vi "21.vi"() -> ()   [LabVIEW 2021]
panel:
  out "Numeric":i32
  out "Array":i32[](array[numeric])
  in  "Number":i32
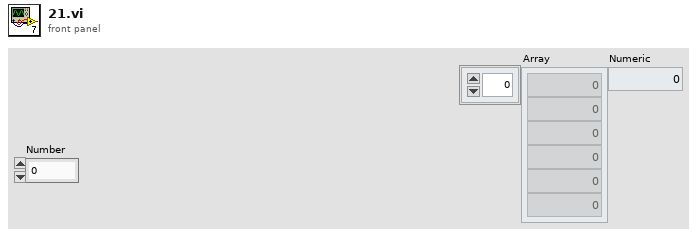
[diagram p1: front panel]
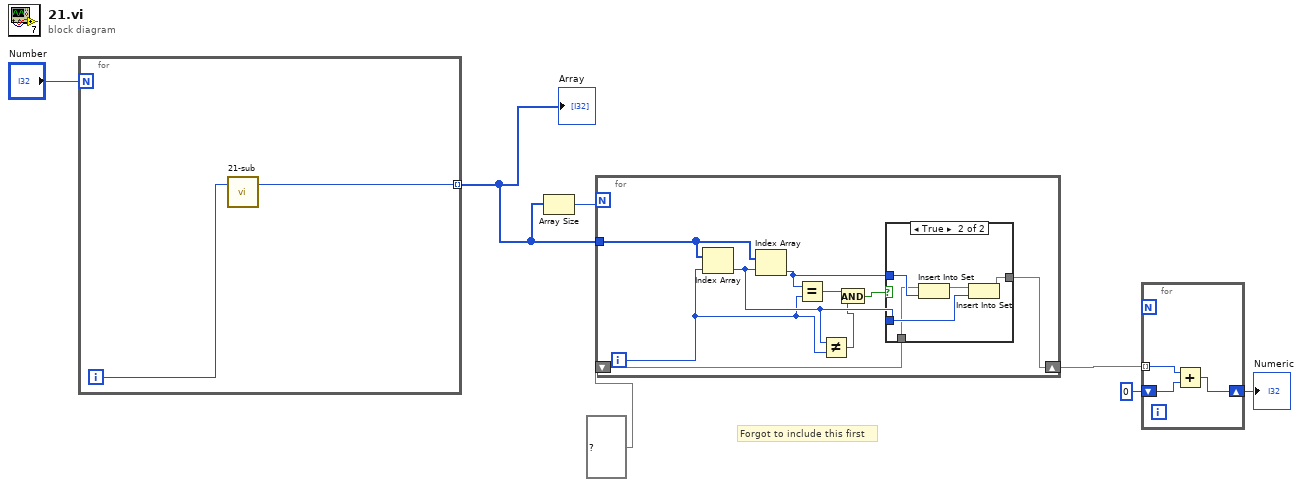
[diagram p0: block diagram]
diagram:
  # "Forgot to include this first"
  n1 = for {
    N: "Number" -> [_]
    tunnel: [w8] -> w5 mode=indexing
    i -> [w9]
    n2 = call "21-sub.vi"("Number"=w9) -> ("Amicable Divisors Sum"=w8:i32)  [unwired: 2 in]
  }
  "Array" <- w5
  n3 = Array Size(array=w5) -> (size(s)=w6:i32)
  n4 = for {
    N: w6 -> [_]
    tunnel: w5 -> [w18]
    shift-right: [w14] -> w3
    shift-left: set{i32} {} ("set in") -> [w15]
    i -> [w11]
    n5 = Index Array(array=w18, index=w11) -> (element=w12:i32)
    n6 = Index Array(array=w18, index=w12) -> (element=w16:i32)
    n7 = Equal?(x=w16, y=w11) -> (x = y?=w17:bool)
    n8 = Not Equal?(x=w12, y=w11) -> (x != y?=w10:bool)
    n9 = And(x=w17, y=w10) -> (x .and. y?=w13:bool)
    n10 = case shown="True" w13 {
      tunnel: w16 -> [_ w24]
      tunnel: w12 -> [_ w22]
      tunnel: w15 -> [w19 w21]
      tunnel: [w19 w20] -> w14
      frame False {
      }
      frame True {
        n11 = Insert Into Set(10:w24, 11:w21) -> (3:w23:set{i32})  [unwired: 1 out]
        n12 = Insert Into Set(10:w22, 11:w23) -> (3:w20:set{i32})  [unwired: 1 out]
      }
    }
  }
  n13 = for {
    tunnel: w3 -> [w27] mode=indexing
    shift-right: [w25] -> w1
    shift-left: 0 -> [w26]
    n14 = Add(x=w27, y=w26) -> (x+y=w25:i32)
  }
  "Numeric" <- w1
